vi "Read Data By File Point.vi"(5 "End Point":i32, 6 "Data Width":i32, 7 "Start Point":i32, 8 "error in":errorcluster, 9 "Skip N Points":i32, 10 "Dimension Size":i32, 11 "Byte Stream File Refnum In":refnum<file>) -> (0 "error out":errorcluster, 2 "Array":sgl[](array[numeric]), 3 "Byte Stream File Refnum Out":refnum<file>)   [LabVIEW 2011, in "Tektronix 7000 Series.lvlib"]
doc: "Reads data between the start and end points from a file."
uses:
  Tektronix 7000 Series.lvlib
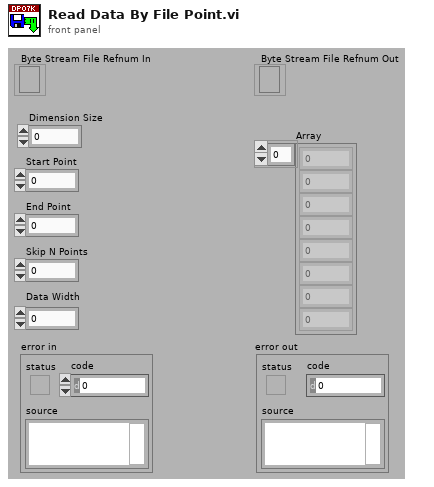
[diagram p1: front panel]
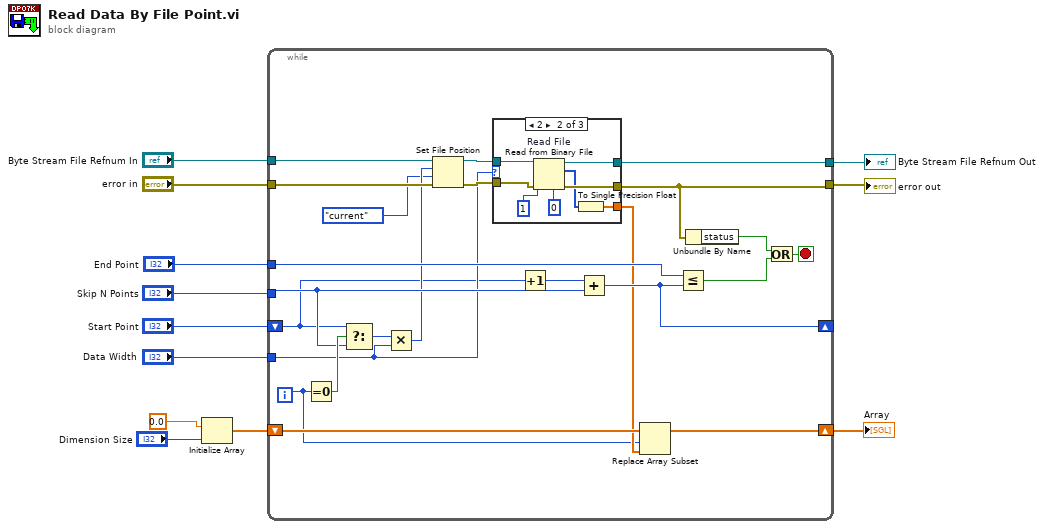
[diagram p0: block diagram]
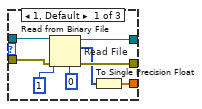
[diagram p2: hidden frame]
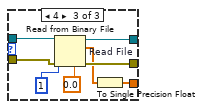
[diagram p3: hidden frame]
diagram:
  n1 = Initialize Array(sgl 0.0 ("element"), "Dimension Size") -> (w3:sgl[])
  n2 = while {
    tunnel: "Byte Stream File Refnum In" -> [w35]
    shift-right: [w30] -> w12
    shift-left: w3 -> [w31]
    tunnel: "Skip N Points" -> [w22]
    shift-right: [w23] -> _
    shift-left: "Start Point" -> [w16]
    tunnel: [w28] -> w9
    tunnel: "End Point" -> [w24]
    tunnel: "error in" -> [w34]
    tunnel: [w25] -> w10
    tunnel: "Data Width" -> [w19]
    i -> [w15]
    stop <- w26 stop-if-true
    n3 = Equal To 0?(x=w15) -> (x = 0?=w29:bool)
    n4 = Select(t=w16, s=w29, f=w22) -> (s? t:f=w21:i32)
    n5 = Multiply(x=w21, y=w19) -> (x*y=w20:i32)
    n6 = Set File Position(offset (in bytes) (0)=w20, refnum=w35, from (0:start)=enum16{"start", "end", "current"}."current" ("pos mode (0:2)"), error in=w34) -> (refnum out=w33:refnum<file>, error out=w32:errorcluster)
    n7 = case shown="2" w19 {
      tunnel: w33 -> [w43 w51 w59]
      tunnel: w32 -> [w42 w50 w58]
      tunnel: [w40 w48 w56] -> w28
      tunnel: [w39 w47 w55] -> w25
      tunnel: [w37 w45 w53] -> w18
      frame 1, Default {
        n8 = Read from Binary File "Read File"(5:i8 0 ("byte stream type"), 8:w42, 10:1 ("count"), 11:w43) -> (0:w39:errorcluster, 2:w36:i8[], 3:w40:refnum<file>)  [unwired: 2 in, 1 out]
        n9 = To Single Precision Float(number=w36) -> (single precision float=w37:sgl[])
      }
      frame 2 {
        n10 = Read from Binary File "Read File"(5:i16 0 ("byte stream type"), 8:w50, 10:1 ("count"), 11:w51) -> (0:w47:errorcluster, 2:w44:i16[], 3:w48:refnum<file>)  [unwired: 2 in, 1 out]
        n11 = To Single Precision Float(number=w44) -> (single precision float=w45:sgl[])
      }
      frame 4 {
        n12 = Read from Binary File "Read File"(5:sgl 0.0 ("byte stream type"), 8:w58, 10:1 ("count"), 11:w59) -> (0:w55:errorcluster, 2:w52:sgl[], 3:w56:refnum<file>)  [unwired: 2 in, 1 out]
        n13 = To Single Precision Float(number=w52) -> (single precision float=w53:sgl[])
      }
    }
    n14 = Increment(x=w16) -> (x+1=w27:i32)
    n15 = Add(x=w27, y=w22) -> (x+y=w23:i32)
    n16 = Replace Array Subset(array=w31, new element=w18, index=w15) -> (w30:sgl[])
    n17 = Less Or Equal?(x=w24, y=w23) -> (x <= y?=w13:bool)
    n18 = Unbundle By Name(w25) -> ("status"=w14:bool)
    n19 = Or(x=w14, y=w13) -> (x .or. y?=w26:bool)
  }
  "Array" <- w12
  "error out" <- w10
  "Byte Stream File Refnum Out" <- w9
